vi "ConvertCropsFromMatlab.vi"(7 "Choose Crop File?":bool, 9 "Crop file":path, 10 "Header In":T2={"header info"={"Header"="", "Head length"=0}, "A/D info"={"# rf points per line"=0, "# lines per scan"=0, "sample rate MHz"=0, "# A/D bits"=0, "# bytes per A/D"=0, "TGC Flag"=0, "A/D Type"=""}, "Tranducer Info"={"bandwidth"=0.0, "center freq"=0.0, "start freq"=0.0, "ID"=0}, "Scan Info"={"delay"=0.0, "pivot distance"=0.0, "sector scan angle"=0.0, "operator"="", "Scan Mode"="", "location"=""}, "Time/Date Info"={"date"="", "time"=""}, "RF Info"={"RF file name"="", "RF file att"="", "RF cal file name"="", "RF cal file att"=""}, "Patient Info"={"ID"="", "extended ID"="", "age"=0, "sex"="", "previously\nscanned"="", "PSA"=0.0, "LOS"=1, "Ethnicty 2"=3, "Race"=3}, "Tissue Type"={"organ"=0, "disease type"=0, "disease location"=0, "IQ_pts"=0, "RcvBuffer"=0, "RcvFrame"=0, "IQBuff"=0, "IQFrame"=0, "IQPage"=0}, "Votage scaling"={"Digitizer (dB)"=0.0, "Gain (dB)"=0.0, "Atten (dB)"=0.0}, "Comment"="", "Misc Info"={"avg num"=0, "c speed"=0, "Div By or SF zones"=0, "XMIT CHS"=0, "RCV CHS"=0, "Xmit angle"=0.0}, "Therapy Parameters"={"Theraputic Freq (MHz)"=0.1, "Time on (s)"=1.0, "Therapy amplitude (mV)"=50.0, "Lines Before"=20, "Lines After"=80}, "Scan Settings"={"Energy (uJ or V)"=0, "Damp (Ohm) or Fc"=0, "HP Filt (KHz)"=0, "LP Filt (MHz)"=0, "Gain (db)"=0, "prf (kHz)"=0.0, "Distance between\nscan lines (um)"=0, "Distance between\nscan planes (um)"=0, "Scan line gap (um)"=0.0, "Scan plane gap (um)"=0.0}, "Compression Parameters"={"F1 (MHz)"=0.0, "F2 (MHz)"=0.0, "% taper"=0.0, "duration"=0.0}, "Patient Info Xtra"={"First Name"="", "Last Name"="", "Notes"=""}, "ROI Box"=[]} {"Compression Parameters"."% taper" min=50 max=1000 format="%.2f"; "Compression Parameters"."F2 (MHz)" format="%.3f"; "Compression Parameters"."F1 (MHz)" format="%.3f"; "Scan Settings"."prf (kHz)" format="%.2f"; "Therapy Parameters"."Therapy amplitude (mV)" min=50 max=1000 format="%.2f"; "Therapy Parameters"."Time on (s)" format="%.3f"; "Therapy Parameters"."Theraputic Freq (MHz)" format="%.3f"; "Patient Info"."Race" items=["Am Ind or Alaska", "Asian", "Hawaiian, Pac Isl", "Black or Afr Amer", "White", "more than one race", "unknown"]; "Patient Info"."Ethnicty 2" items=["Hispanic", "Non-Hispanic", "unknown"]; "Patient Info"."LOS" items=["1", "2", "3", "4", "5"]; "Patient Info"."PSA" format="%.1f"; "Scan Info"."delay" format="%.2f"; "Scan Info"."pivot distance" format="%.2f"; "Scan Info"."sector scan angle" format="%.2f"; "Tranducer Info"."bandwidth" format="%.2f"; "Tranducer Info"."center freq" format="%.2f"; "Tranducer Info"."start freq" format="%.2f"}, 11 "Directory":path=path "\\\\vantage-n-wk\\Vantage Data/Adam Doppler/2016-08-12/HFR_03A_20D_08kHz_16MHz_00_EYE") -> (3 "crop marks":T1)   [LabVIEW 2022 SP3]
uses:
  ViewData/-ReadEye/Header.ctl
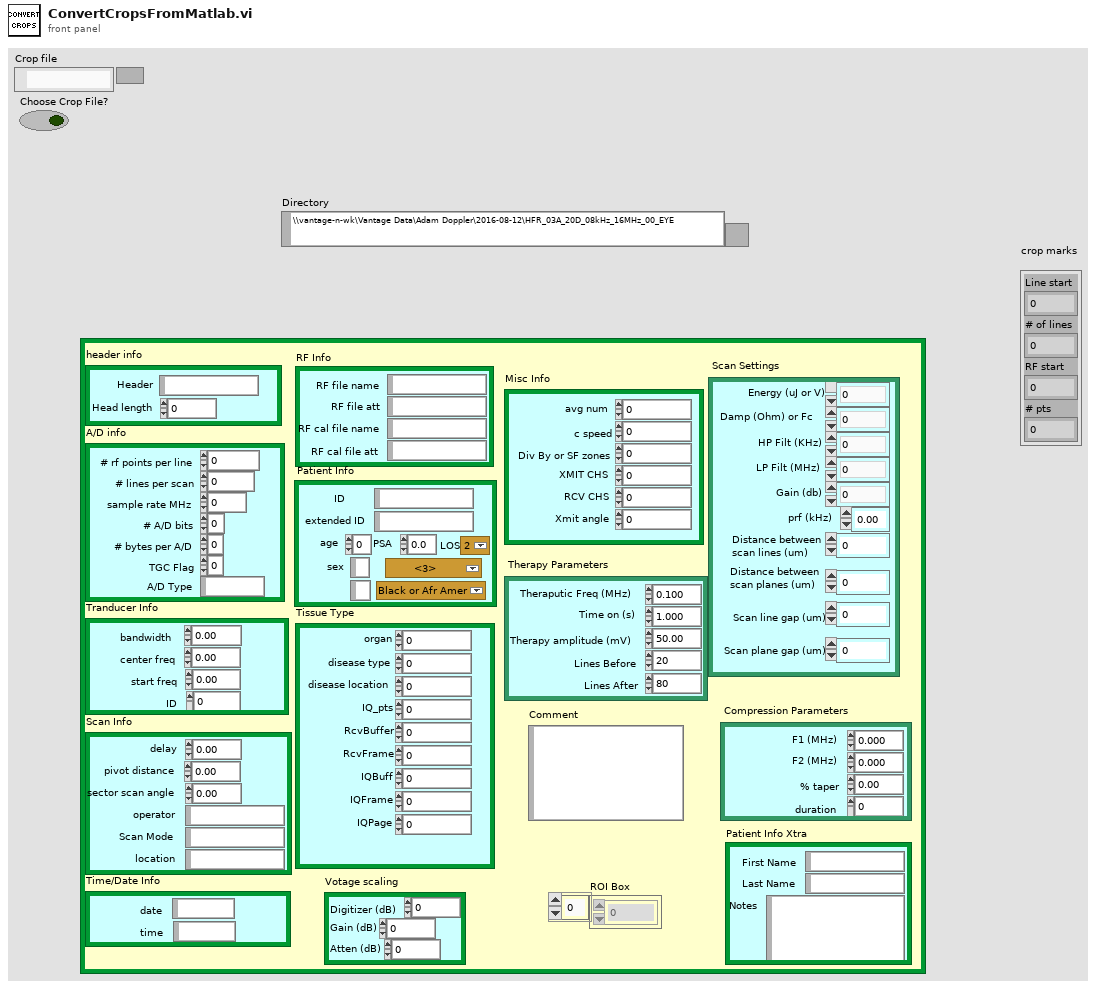
[diagram p1: front panel]
types:
  T1 = cluster{"Line start":dbl, "# of lines":dbl, "RF start":dbl, "# pts":dbl}
  T2 = typedef "Header.ctl" = cluster{"header info":cluster{"Header":string, "Head length":i16}, "A/D info":cluster{"# rf points per line":u16, "# lines per scan":u16, "sample rate MHz":u16, "# A/D bits":i16, "# bytes per A/D":u16, "TGC Flag":u16, "A/D Type":string}, "Tranducer Info":cluster{"bandwidth":sgl, "center freq":sgl, "start freq":sgl, "ID":i32}, "Scan Info":cluster{"delay":sgl, "pivot distance":sgl, "sector scan angle":sgl, "operator":string, "Scan Mode":string, "location":string}, "Time/Date Info":cluster{"date":string, "time":string}, "RF Info":cluster{"RF file name":string, "RF file att":string, "RF cal file name":string, "RF cal file att":string}, "Patient Info":cluster{"ID":string, "extended ID":string, "age":u16, "sex":string, "previously\nscanned":string, "PSA":sgl, "LOS":u8, "Ethnicty 2":u8, "Race":u8}, "Tissue Type":cluster{"organ":i16, "disease type":i16, "disease location":i16, "IQ_pts":u16, "RcvBuffer":u8, "RcvFrame":u16, "IQBuff":u8, "IQFrame":u16, "IQPage":u8}, "Votage scaling":cluster{"Digitizer (dB)":sgl, "Gain (dB)":sgl, "Atten (dB)":sgl}, "Comment":string, "Misc Info":cluster{"avg num":u16, "c speed":i16, "Div By or SF zones":i16, "XMIT CHS":u8, "RCV CHS":u8, "Xmit angle":sgl}, "Therapy Parameters":cluster{"Theraputic Freq (MHz)":sgl, "Time on (s)":sgl, "Therapy amplitude (mV)":sgl, "Lines Before":u16, "Lines After":u16}, "Scan Settings":cluster{"Energy (uJ or V)":u8, "Damp (Ohm) or Fc":u8, "HP Filt (KHz)":u8, "LP Filt (MHz)":u8, "Gain (db)":u8, "prf (kHz)":sgl, "Distance between\nscan lines (um)":u16, "Distance between\nscan planes (um)":u16, "Scan line gap (um)":sgl, "Scan plane gap (um)":sgl}, "Compression Parameters":cluster{"F1 (MHz)":sgl, "F2 (MHz)":sgl, "% taper":sgl, "duration":sgl}, "Patient Info Xtra":cluster{"First Name":string, "Last Name":string, "Notes":string}, "ROI Box":u16[]}
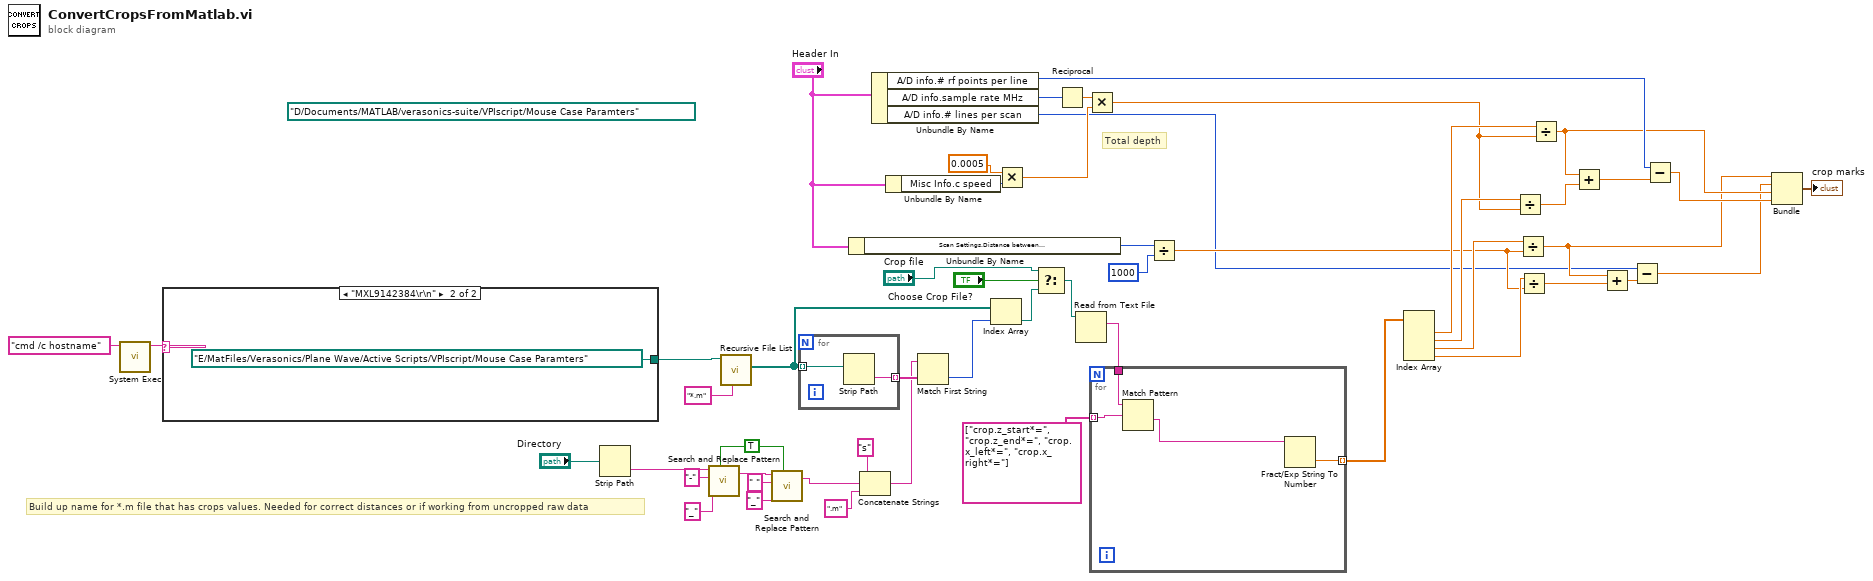
[diagram p0: block diagram]
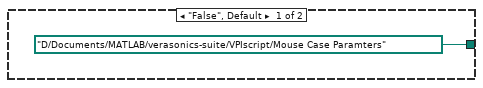
[diagram p2: hidden frame]
diagram:
  (unwired) path "D:/Documents/MATLAB/verasonics-suite/VPIscript/Mouse Case Paramters"
  w39 = TRUE ("replace all? (F)")
  # "Build up name for *.m file that has crops values. Needed for correct distances or if working from uncropped raw data"
  # "Total depth"
  n1 = call <vilib>:"System Exec.vi"("command line"="cmd /c hostname") -> ("standard output"=w7:string)  [unwired: 7 in, 3 out]
  n2 = case shown="\"MXL9142384\\r\\n\"" w7 {
    tunnel: [path "D:/Documents/MATLAB/verasonics-suite/VPIscript/Mouse Case Paramters" path "E:/MatFiles/Verasonics/Plane Wave/Active Scripts/VPIscript/Mouse Case Paramters"] -> w6
    frame "False", Default {
    }
    frame "MXL9142384\r\n" {
    }
  }
  n3 = Strip Path(path="Directory") -> (name=w51:string)  [unwired: 1 out]
  n4 = call <vilib>:"Search and Replace Pattern.vi"("string"=w51, "regular expression (\"\")"="-" ("regular expression (\"\")"), "replace string (\"\")"="_" ("replace string (\"\")"), "replace all? (F)"=w39) -> ("result string"=w42:string)  [unwired: 1 in, 1 out]
  n5 = call <vilib>:"Recursive File List.vi"("pattern"="*.m", "Folder Path"=w6) -> ("All Files in Dir"=w37:path[])  [unwired: 5 in, 4 out]
  n6 = call <vilib>:"Search and Replace Pattern.vi"("string"=w42, "regular expression (\"\")"=" " ("regular expression (\"\")"), "replace string (\"\")"="_" ("replace string (\"\")"), "replace all? (F)"=w39) -> ("result string"=w41:string)  [unwired: 1 in, 1 out]
  n7 = for {
    tunnel: w37 -> [w55] mode=indexing
    tunnel: [w54] -> w45 mode=indexing
    n8 = Strip Path(path=w55) -> (name=w54:string)  [unwired: 1 out]
  }
  n9 = Unbundle By Name("Header In") -> ("Scan Settings.Distance between\nscan lines (um)"=w31:u16)
  n10 = Concatenate Strings("s" ("string"), w41, ".m" ("string")) -> (w44:string)
  n11 = Unbundle By Name("Header In") -> ("A/D info.# rf points per line"=w23:u16, "A/D info.sample rate MHz"=w32:u16, "A/D info.# lines per scan"=w12:u16)
  n12 = Unbundle By Name("Header In") -> ("Misc Info.c speed"=w30:i16)
  n13 = Match First String(2:w45, 3:w44) -> (0:w38:i32)  [unwired: 1 out]
  n14 = Index Array(array=w37, index=w38) -> (element=w2:path)
  n15 = Multiply(x=0.0005, y=w30) -> (x*y=w28:dbl)
  n16 = Select(t="Crop file", s="Choose Crop File?", f=w2) -> (s? t:f=w4:path)
  n17 = Reciprocal(x=w32) -> (1/x=w33:dbl)
  n18 = Read from Text File(file (use dialog)=w4) -> (text=w36:string)  [unwired: 3 in, 3 out]
  n19 = Multiply(x=w33, y=w28) -> (x*y=w24:dbl)
  n20 = for {
    tunnel: w36 -> [w59]
    tunnel: string[] ["crop.z_start*=", "crop.z_end*=", "crop.x_left*=", "crop.x_right*="] -> [w57] mode=indexing
    tunnel: [w56] -> w27 mode=indexing
    n21 = Match Pattern(string=w59, regular expression=w57) -> (after substring=w58:string)  [unwired: 1 in, 3 out]
    n22 = Fract/Exp String To Number(string=w58) -> (number=w56:dbl)  [unwired: 3 in, 1 out]
  }
  n23 = Divide(x=w31, y=1000) -> (x/y=w18:dbl)
  n24 = Index Array(array=w27) -> (element #1=w26:dbl, element #2=w25:dbl, element #3=w20:dbl, element #4=w19:dbl)  [unwired: 4 in]
  n25 = Divide(x=w25, y=w24) -> (x/y=w22:dbl)
  n26 = Divide(x=w20, y=w18) -> (x/y=w14:dbl)
  n27 = Divide(x=w19, y=w18) -> (x/y=w13:dbl)
  n28 = Divide(x=w26, y=w24) -> (x/y=w17:dbl)
  n29 = Add(x=w17, y=w22) -> (x+y=w21:dbl)
  n30 = Add(x=w14, y=w13) -> (x+y=w15:dbl)
  n31 = Subtract(x=w12, y=w15) -> (x-y=w11:dbl)
  n32 = Subtract(x=w23, y=w21) -> (x-y=w16:dbl)
  n33 = Bundle(w14, w11, w17, w16) -> (→"crop marks":cluster{dbl, dbl, dbl, dbl})  [unwired: 1 in]
